vi "ChangeStateJumpToError.vi"(8 "err in":errorcluster, 11 "Next State (pre error check)":T1=enum."Play File") -> (0 "err out":errorcluster, 3 "Next State (post error check)":T1=enum."Play File")   [LabVIEW 2017]
uses:
  TypeDef/RF_StateMachine.ctl
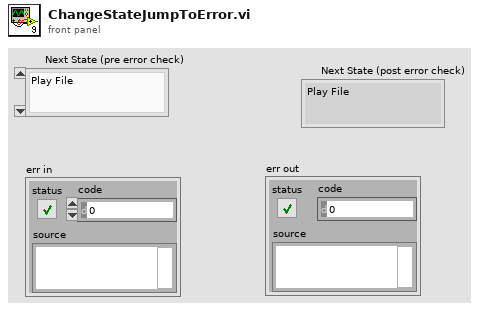
[diagram p1: front panel]
types:
  T1 = typedef "RF_StateMachine.ctl" = enum16{"Parse Metadata", "Convert File", "Play File", "Finished Playing", "Send Message", "Report Error", "Exit"}
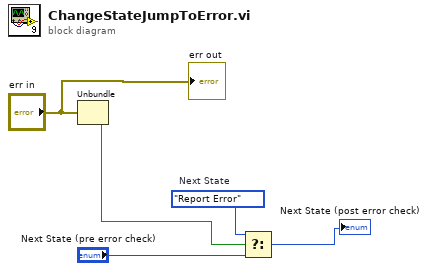
[diagram p0: block diagram]
diagram:
  w4 = RF_StateMachine."Report Error"  # Next State
  n1 = Unbundle("err in") -> ("status"=w5:bool)  [unwired: 2 out]
  n2 = Select(t=w4, s=w5, f="Next State (pre error check)") -> (s? t:f=→"Next State (post error check)":T1)
  "err out" <- "err in"
